vi "roi divisible by 4.vi"(11 "ROI Descriptor Out":T1) -> (1 "floor(x/y) 2":i32, 2 "floor(x/y)":i32)   [LabVIEW 2013]
panel:
  out "height":i32
  out "width":i32
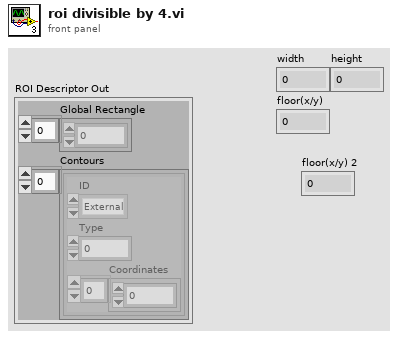
[diagram p1: front panel]
types:
  T1 = cluster{"Global Rectangle":i32[], "Contours":cluster{"ID":enum32{"External", "Internal"}, "Type":u32, "Coordinates":i32[]}[]}
  T2 = cluster{"ID":enum32{"External", "Internal"}, "Type":u32, "Coordinates":i32[]}[]
  T3 = cluster{"ID":enum32{"External", "Internal"}, "Type":u32, "Coordinates":i32[]}
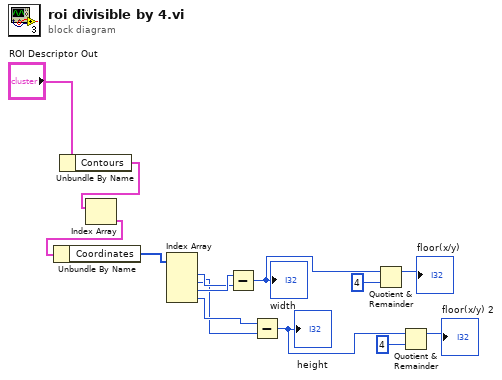
[diagram p0: block diagram]
diagram:
  n1 = Unbundle By Name("ROI Descriptor Out") -> ("Contours"=w13:T2)
  n2 = Index Array(array=w13) -> (element=w14:T3)  [unwired: 1 in]
  n3 = Unbundle By Name(w14) -> ("Coordinates"=w11:i32[])
  n4 = Index Array(array=w11) -> (element #1=w9:i32, element #2=w7:i32, element #3=w10:i32, element #4=w8:i32)  [unwired: 4 in]
  n5 = Subtract(x=w10, y=w9) -> (x-y=w6:i32)
  "width" <- w6
  n6 = Subtract(x=w8, y=w7) -> (x-y=w1:i32)
  "height" <- w1
  n7 = Quotient & Remainder(x=w6, y=4) -> (x-y*floor(x/y)=→"floor(x/y)":i32)  [unwired: 1 out]
  n8 = Quotient & Remainder(x=w1, y=4) -> (x-y*floor(x/y)=→"floor(x/y) 2":i32)  [unwired: 1 out]
